vi "WriteJSON.vi"(2 "error in (no error)":errorcluster, 3 "JSONEventInfo":variant) -> (1 "test case exists?":bool)   [LabVIEW 2018]
uses:
  <vilib>/LVH/i3 JSON/JSON Parsing/Get Object Parameter Files/Get Object Parameter - String.vi
  Global Variables.vi
  <vilib>/LVH/i3 JSON/JSON Generation/Create Value Files/Create Value - Object.vi
  <vilib>/LVH/i3 JSON/JSON Generation/Add Object Parameter Files/Add Object Parameter - Object.vi
  <vilib>/LVH/i3 JSON/JSON Generation/Add Object Parameter Files/Add Object Parameter - String.vi
  <vilib>/LVH/i3 JSON/JSON Generation/Append to Array Files/Append to Array - Object.vi
  <vilib>/LVH/i3 JSON/i3-json.lvlib
panel:
  out "is JSON Null?":bool
  out "JSONpath":path
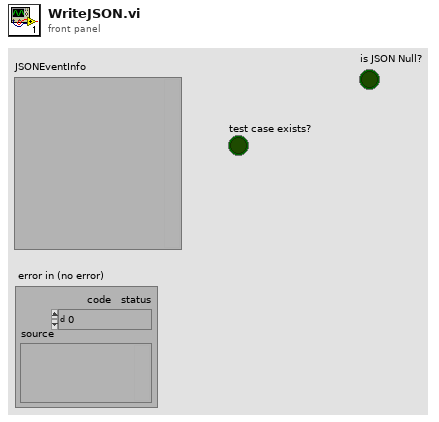
[diagram p1: front panel]
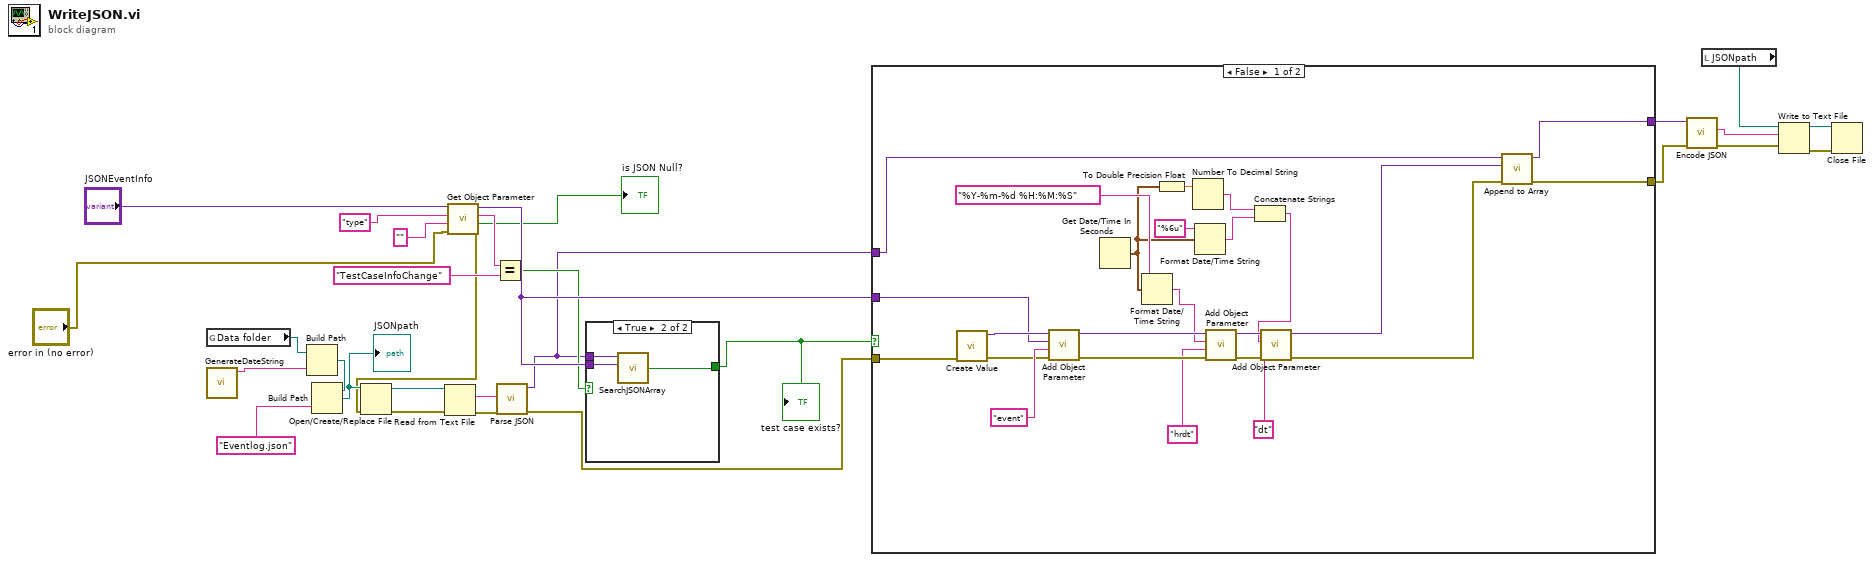
[diagram p0: block diagram]
diagram:
  n1 = global read "Global Variables.vi" "Data folder"() -> (w28:path)
  n2 = call "GenerateDateString.vi"() -> ("String"=w29:string)  [unwired: 11 in]
  n3 = Build Path(base path=w28, name or relative path=w29) -> (appended path=w27:path)
  n4 = Build Path(base path=w27, name or relative path="Eventlog.json" ("string")) -> (appended path=w21:path)
  "JSONpath" <- w21
  n5 = call-poly <vilib>:"Get Object Parameter.vi"("error in (no error)"="error in (no error)", "Default Value if JSON Null"="", "Parameter Name"="type" ("Default Value if JSON Null"), "JSON Tree In (JSON Object)"="JSONEventInfo") -> ("error out"=w1:errorcluster, "is JSON Null?"=→"is JSON Null?":bool, "String Value"=w17:string, "JSON Tree Out Passthrough"=w20:variant)  [unwired: 4 in]
  n6 = Open/Create/Replace File(file path (use dialog)=w21, error in=w1) -> (refnum out=w25:refnum<file>, error out=w22:errorcluster)  [unwired: 4 in, 1 out]
  n7 = Read from Text File(file (use dialog)=w25, error in=w22) -> (text=w23:string, error out=w24:errorcluster)  [unwired: 2 in, 2 out]
  n8 = Equal?(x=w17, y="TestCaseInfoChange") -> (x = y?=w18:bool)
  n9 = call <vilib>:"Parse JSON.vi"("error in (no error)"=w24, "JSON String"=w23) -> ("error out"=w8:errorcluster, "JSON Tree"=w14:variant)  [unwired: 6 in, 2 out]
  n10 = case shown="True" w18 {
    selector: w18 -> [w30 _]
    tunnel: w14 -> [_ w33]
    tunnel: w20 -> [_ w32]
    tunnel: [w30 w31] -> w15
    frame False {
    }
    frame True {
      n11 = call "SearchJSONArray.vi"("eventinfoJSON"=w32, "JSONArray"=w33) -> ("Boolean"=w31:bool)  [unwired: 4 in]
    }
  }
  "test case exists?" <- w15
  n12 = case shown="False" w15 {
    tunnel: w20 -> [w40 _]
    tunnel: w14 -> [w38 w59]
    tunnel: [w36 w58] -> w6
    tunnel: [w35 w59] -> w9
    tunnel: w8 -> [w34 w58]
    frame False {
      n13 = call-poly <vilib>:"Create Value.vi"("error in (no error)"=w34) -> ("error out"=w41:errorcluster, "JSON Tree"=w42:variant)  [unwired: 9 in]
      n14 = call-poly <vilib>:"Add Object Parameter.vi"("error in (no error)"=w41, "Name"="event", "JSON Object"=w40, "JSON Tree in (JSON Object)"=w42) -> ("error out"=w56:errorcluster, "JSON Tree out (JSON Object)"=w57:variant)  [unwired: 6 in]
      n15 = Get Date/Time In Seconds() -> (seconds since 1Jan1904=w48:timestamp)
      n16 = Format Date/Time String(time format string (%c)="%Y-%m-%d %H:%M:%S", seconds (now)=w48) -> (date/time string=w52:string)  [unwired: 1 in]
      n17 = To Double Precision Float(number=w48) -> (double precision float=w47:dbl)
      n18 = Number To Decimal String(number=w47) -> (decimal integer string=w49:string)  [unwired: 1 in]
      n19 = Format Date/Time String(time format string (%c)="%6u", seconds (now)=w48) -> (date/time string=w50:string)  [unwired: 1 in]
      n20 = call-poly <vilib>:"Add Object Parameter.vi"("error in (no error)"=w56, "Name"="hrdt", "String"=w52, "JSON Tree in (JSON Object)"=w57) -> ("error out"=w45:errorcluster, "JSON Tree out (JSON Object)"=w46:variant)  [unwired: 6 in]
      n21 = Concatenate Strings(w49, w50) -> (w43:string)
      n22 = call-poly <vilib>:"Add Object Parameter.vi"("error in (no error)"=w45, "Name"="dt", "String"=w43, "JSON Tree in (JSON Object)"=w46) -> ("error out"=w37:errorcluster, "JSON Tree out (JSON Object)"=w39:variant)  [unwired: 6 in]
      n23 = call-poly <vilib>:"Append to Array.vi"("error in (no error)"=w37, "JSON Object"=w39, "JSON Tree in (JSON Array)"=w38) -> ("error out"=w36:errorcluster, "JSON Tree out (JSON Array)"=w35:variant)  [unwired: 7 in]
    }
    frame True {
    }
  }
  n24 = call <vilib>:"Encode JSON.vi"("error in (no error)"=w6, "JSON Tree"=w9) -> ("error out"=w13:errorcluster, "String"=w10:string)  [unwired: 4 in]
  n25 = local read "JSONpath"() -> (w7:path)
  n26 = Write to Text File(file (use dialog)=w7, text=w10, error in=w13) -> (refnum out=w11:refnum<file>, error out=w12:errorcluster)  [unwired: 1 in, 1 out]
  n27 = Close File(refnum=w11, error in=w12) -> ()  [unwired: 2 out]
